vi "Keepalive.vi"(8 "error in (no error)":errorcluster, 10 "IPv4 Endpoint":T1, 11 "Telemetry Server in":refnum<class "Telemetry Server.lvclass">) -> (0 "error out":errorcluster, 3 "Telemetry Server out":refnum<class "Telemetry Server.lvclass">)   [LabVIEW 2020, in "VolatusTelemetry.lvlib" / "Telemetry Server.lvclass"]
uses:
  Telemetry Server.lvclass
  Telemetry Server.lvclass/Telemetry Server.ctl
  IPv4 Endpoint.ctl
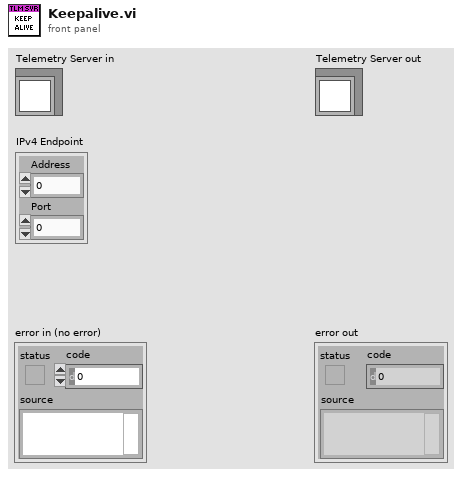
[diagram p1: front panel]
types:
  T1 = typedef "VolatusTelemetry.lvlib/Telemetry Server.lvclass/IPv4 Endpoint.ctl" = cluster{"Address":u32, "Port":u16}
  T2 = typedef "VolatusTelemetry.lvlib/Telemetry Server.lvclass/Client Info.ctl" = cluster{"Node":string, "Alias":string, "Keepalive Time":dbl}
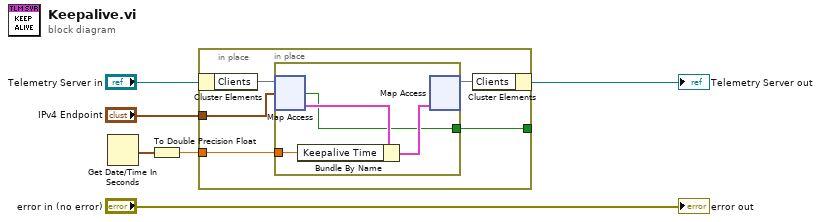
[diagram p0: block diagram]
diagram:
  n1 = Get Date/Time In Seconds() -> (seconds since 1Jan1904=w5:timestamp)
  n2 = To Double Precision Float(number=w5) -> (double precision float=w3:dbl)
  n3 = in-place {
    in-place-border: w3 -> [w9]
    in-place-border: "IPv4 Endpoint" -> [w10]
    in-place-border: [w7] -> _
    n4 = in-place-cluster #1("Telemetry Server in") -> ("Clients"=w11:map{T1, T2})
    n5 = in-place {
      in-place-border: w9 -> [w14]
      in-place-border: [w12] -> w7
      n6 = in-place-map #2(w11, w10) -> (w15:T2, w12:bool)  [unwired: 1 in]
      n7 = Bundle By Name(cluster=w15, "Keepalive Time"=w14) -> (w13:T2)
      n8 = in-place-map #2(w13) -> (w8:map{T1, T2})  [unwired: 1 in, 2 out]
    }
    n9 = in-place-cluster #1("Clients"=w8) -> (→"Telemetry Server out":refnum<class "Telemetry Server.lvclass">)
  }
  "error out" <- "error in (no error)"
